vi "DB select data(index).vi"(6 "index":i32, 7 "Condtion":string, 8 "error in (no error)":errorcluster caption="错误输入（无错误）", 9 "Code":string, 10 "Tabe":string, 11 "Connncet State":T1) -> (0 "error out":errorcluster caption="错误输出", 1 "state":bool, 2 "data":variant[][](array[variant]), 3 "Connncet State out":T1)   [LabVIEW 2014]
uses:
  <vilib>/addons/database/NI_Database_API.lvlib
  Ctr/Constr.ctl
  <vilib>/addons/database/Connection.llb/Conn ObjectReference.ctl
  Ctr/Conneect State.ctl
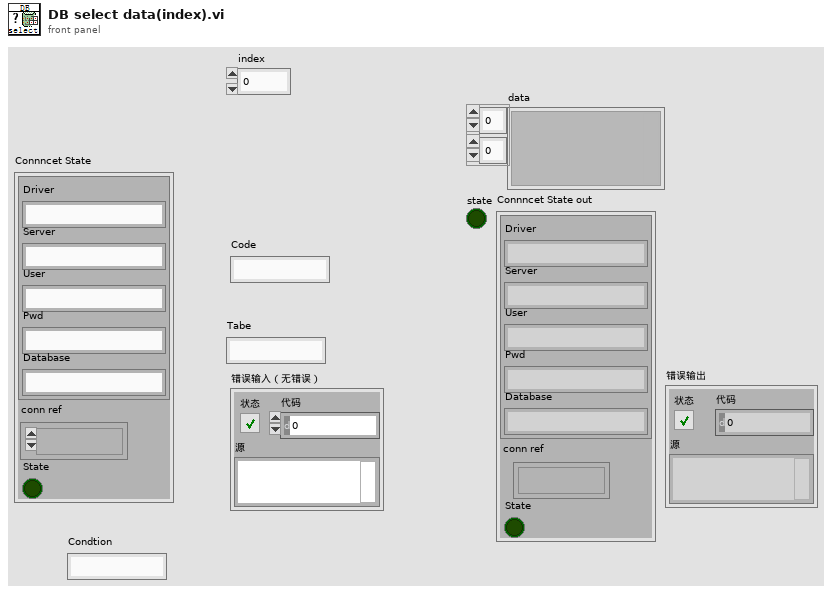
[diagram p1: front panel]
types:
  T1 = typedef "Conneect State.ctl" = cluster{"Constr":T2, "conn ref":T3, "State":bool}
  T2 = typedef "Constr.ctl" = cluster{"Driver":string, "Server":string, "User":string, "Pwd":string, "Database":string}
  T3 = typedef "NI_Database_API.lvlib/Conn ObjectReference.ctl" = refnum<k1>
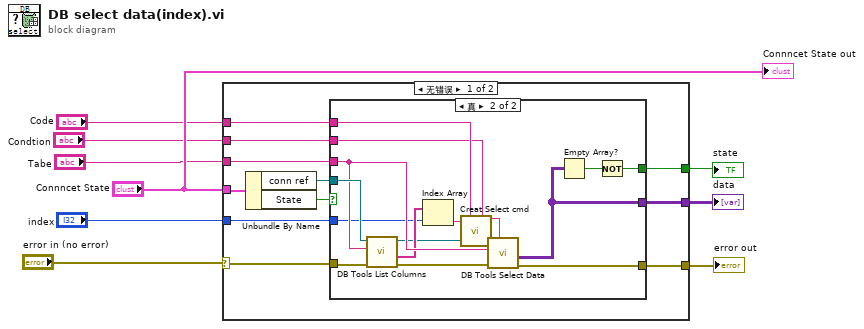
[diagram p0: block diagram]
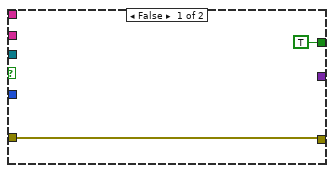
[diagram p2: hidden frame]
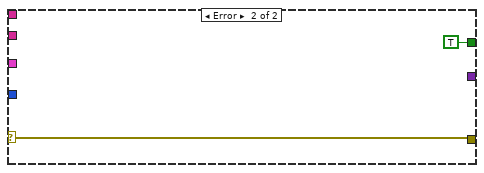
[diagram p3: hidden frame]
diagram:
  n1 = case shown="无错误" "error in (no error)" {
    selector: "error in (no error)" -> [w18 w39]
    tunnel: "Connncet State" -> [w20 _]
    tunnel: "Tabe" -> [w16 _]
    tunnel: "Code" -> [w15 _]
    tunnel: [w14 w39] -> w5
    tunnel: [w13 _] -> w4
    tunnel: [w12 TRUE] -> w3
    tunnel: "index" -> [w11 _]
    tunnel: "Condtion" -> [w10 _]
    frame No Error {
      n2 = Unbundle By Name(w20) -> ("conn ref"=w17:T3, "State"=w19:bool)
      n3 = case shown="真" w19 {
        tunnel: w18 -> [w22 w33]
        tunnel: w17 -> [_ w32]
        tunnel: w16 -> [_ w31]
        tunnel: w15 -> [_ w29]
        tunnel: [w22 w37] -> w14
        tunnel: [_ w36] -> w13
        tunnel: [TRUE w34] -> w12
        tunnel: w11 -> [_ w24]
        tunnel: w10 -> [_ w23]
        frame False {
        }
        frame True {
          n4 = call <vilib>:"DB Tools List Columns.vi"("error in (no error)"=w33, "table"=w31, "connection reference"=w32) -> ("error out"=w30:errorcluster, "columns"=w27:string[], "connection reference out"=w26:T3)  [unwired: 1 in, 1 out]
          n5 = Index Array(array=w27, index=w24) -> (element=w25:string)
          n6 = call "Creat Select cmd.vi"("Col"=w25, "Code"=w29, "Condtion"=w23) -> ("Str"=w28:string)  [unwired: 11 in, 1 out]
          n7 = call <vilib>:"DB Tools Select Data.vi"("condition"=w28, "error in (no error)"=w30, "table"=w31, "connection reference"=w26) -> ("error out"=w37:errorcluster, "data"=w36:variant[][])  [unwired: 2 in, 1 out]
          n8 = Empty Array?(array=w36) -> (empty?=w35:bool)
          n9 = Not(x=w35) -> (.not. x?=w34:bool)
        }
      }
    }
    frame Error {
    }
  }
  "error out" <- w5
  "data" <- w4
  "state" <- w3
  "Connncet State out" <- "Connncet State"
